vi "AdvancedProgram.vi"() -> ()   [LabVIEW 2018, in "JULABO DeviceDriver.lvlib"]
doc: "Advanced event triggered example"
uses:
  JULABO DeviceDriver.lvlib
panel:
  out "device error out":errorcluster
  out "error out 2":errorcluster caption="error out"
  out "error out":errorcluster
  in  "Registerkartenelement":T1(tab)
  out "Safetytemp":dbl
  out "ExcessTempProtection":dbl
  in  "Control":enum16{"Internal", "External"}(ring)
  out "ExternalTemp":dbl format="%.2f"
  in  "Setpoint":dbl format="%.2f"
  out "InternalTemp":dbl format="%.2f"
  out "Power":i8(slide) scale=-100.0..100.0
  out "Diagram":T2(graph)
  in  "StartStop":bool
  in  "btnAdjustInternalTempLimits":bool
  in  "btnAdjustBandLimits":bool
  in  "btnAdjustCapacityLevels":bool
  in  "btnAdjustWarningLevels":bool
  in  "Upper Bandlimit":dbl=100.0 min=0.0 max=200.0
  in  "Lower Bandlimit":dbl min=0.0 max=200.0
  in  "InternMin":dbl format="%.2f"
  in  "InternMax":dbl=50.0 format="%.2f"
  in  "CoolMax":i8=-100 min=-100 max=0
  in  "HeatMax":u8=50 max=100
  in  "Subtemp":dbl=-20.0 format="%.2f"
  in  "Overtemp":dbl=50.0 format="%.2f"
  in  "Tv (0s) 2":u16 max=999
  in  "Tn (3s) 2":u16=3 min=3 max=9999
  in  "Xp (0.6K) 2":dbl=0.6 min=0.1 max=99.9
  in  "btnAdjustExternalControlParams":bool
  in  "XpU (0.6K)":dbl=0.6 min=0.1 max=99.9
  in  "Dynamic (0: aperiodic)":enum16{"aperiodic", "standard"}(ring)
  in  "btnAdjustInternalControlParams":bool
  in  "Tv (0s)":u16 max=999
  in  "Tn (3s)":u16=3 min=3 max=9999
  in  "Xp (0.6K)":dbl=0.6 min=0.1 max=99.9
  in  "ReadCycle":i32=1000
  in  "Stopp":bool
  in  "ID Query? (T: Yes)":bool=TRUE
  in  "RS485-Address (128: RS232)":u32=128
  in  "VISA resource name":refnum<visa-resource-name>="COM3"
  in  "Serial Configuration":T3={"Baud Rate"=4800, "Parity"=2, "Data Bits"=7, "Stop Bits"=10, "Flow Control"=2} {"Flow Control" items=["None", "XON/XOFF", "RTS/CTS", "XON/XOFF & RTS/CTS", "DTR/DSR", "XON/XOFF & DTR/DSR"]; "Stop Bits" items=["1.0"=10, "1.5"=15, "2.0"=20]; "Data Bits" items=["7"=7, "8"=8]; "Parity" items=["None", "Odd", "Even", "Mark", "Space"]; "Baud Rate" items=["300"=300, "600"=600, "1200"=1200, "2400"=2400, "4800"=4800, "9600"=9600, "19200"=19200]}
  in  "Reset / Default (T: Both)":bool=TRUE
  # "1. Select the COM-Port and adjust the serial\nconfiguration for your instrument\n2. Adjust the Read cycle\n3. Start the VI by pressing the \"Start\" -Button\n( Arrow button on the top-left corner)\n4. To stop the execution press the \"Stop\" button"
  # "Internal parameters"
  # "External parameters"
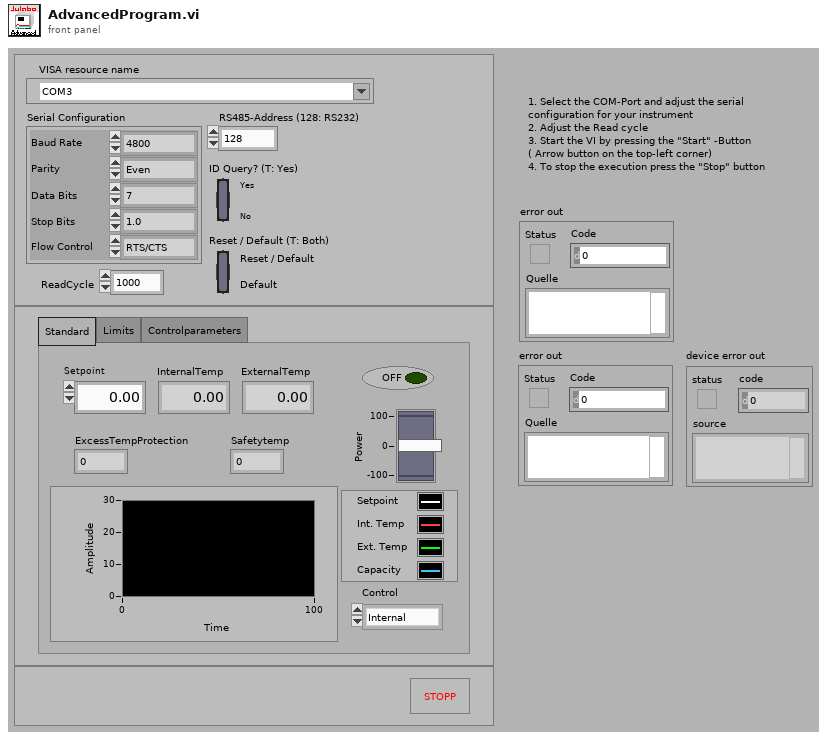
[diagram p1: front panel]
types:
  T1 = enum32{"Standard", "Limits", "Controlparameters"}
  T2 = cluster{"Setpoint (out)":dbl, "InternalTemp (out)":dbl, "ExternalTemp (out)":dbl, "Capacity (out)":i8}
  T3 = cluster{"Baud Rate":u32, "Parity":u16, "Data Bits":u16, "Stop Bits":u16, "Flow Control":u16}
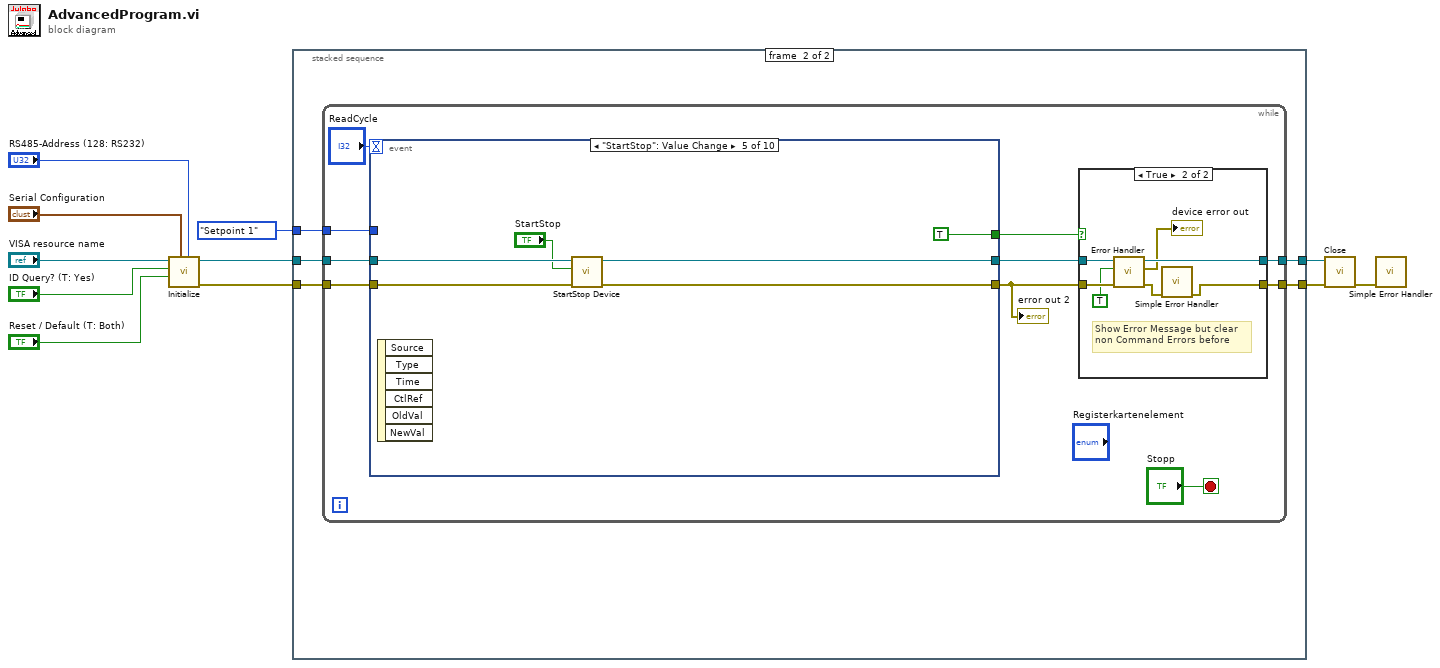
[diagram p0: block diagram]
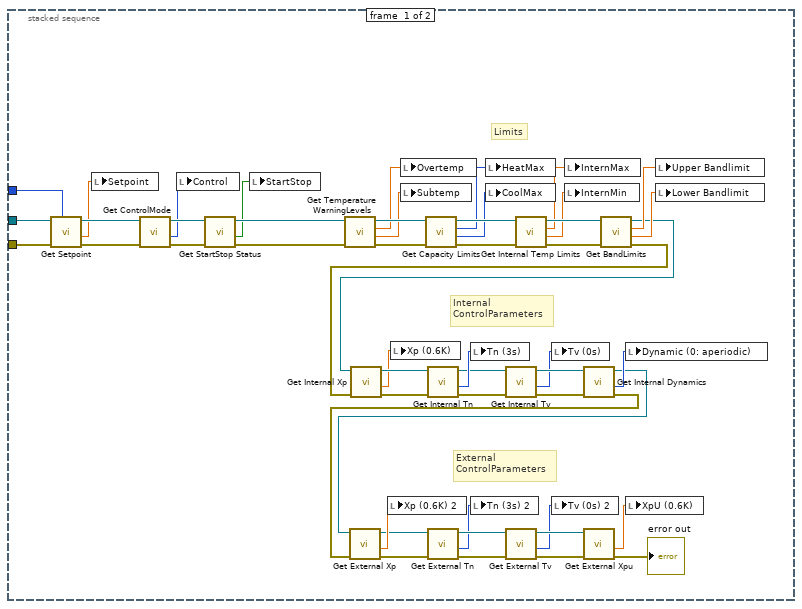
[diagram p2: hidden frame]
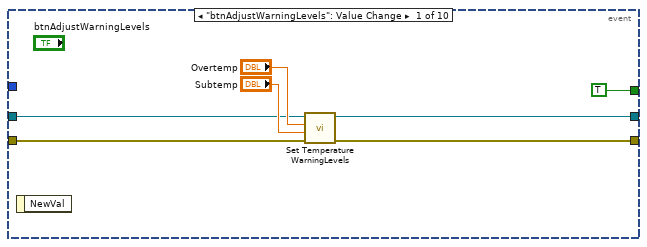
[diagram p4: hidden frame]
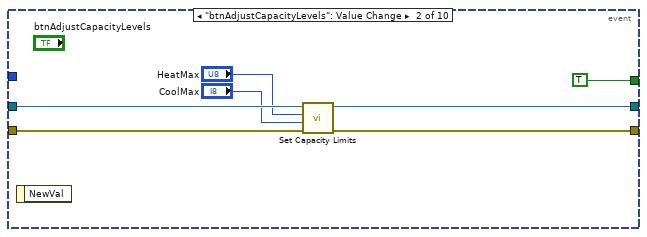
[diagram p5: hidden frame]
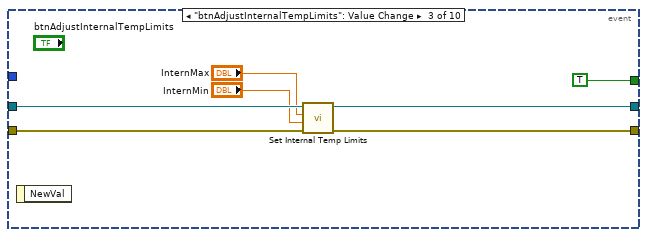
[diagram p6: hidden frame]
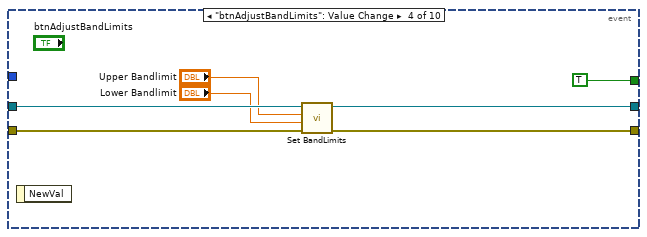
[diagram p7: hidden frame]
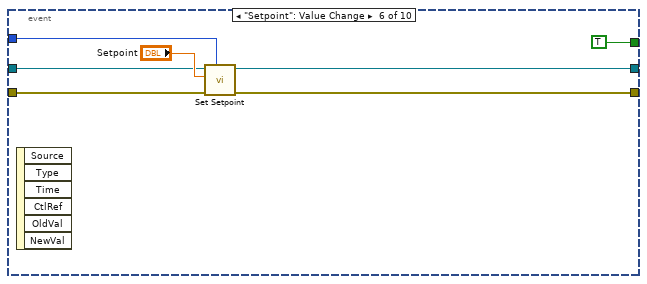
[diagram p8: hidden frame]
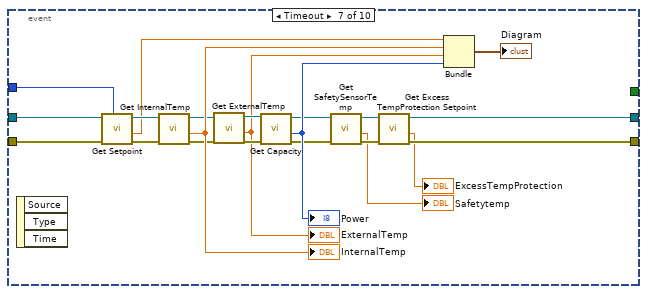
[diagram p9: hidden frame]
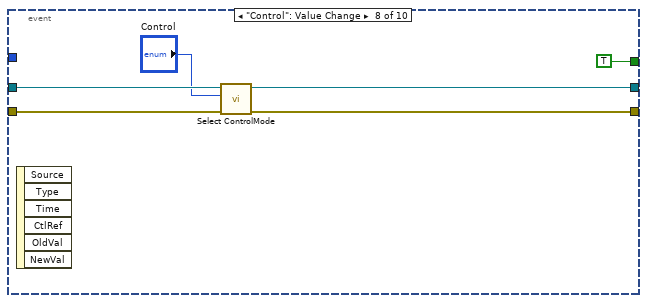
[diagram p10: hidden frame]
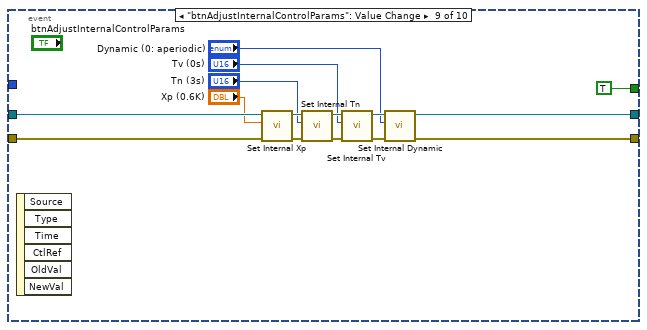
[diagram p11: hidden frame]
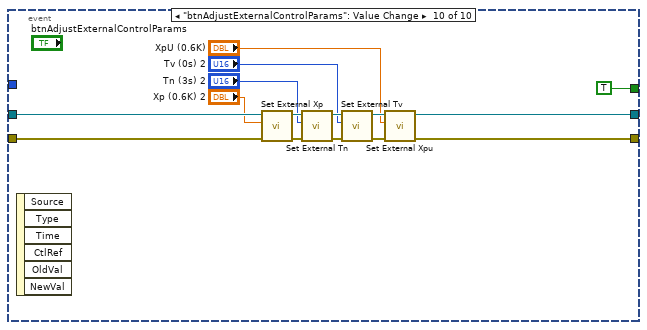
[diagram p12: hidden frame]
diagram:
  n1 = call "Initialize.vi"("RS485-Address (128: RS232)"="RS485-Address (128: RS232)", "Serial Configuration"="Serial Configuration", "Reset / Default (T: Both)"="Reset / Default (T: Both)", "ID Query? (T: Yes)"="ID Query? (T: Yes)", "VISA resource name"="VISA resource name") -> ("error out"=w4:errorcluster, "VISA resource name out"=w5:refnum<visa-resource-name>)  [unwired: 5 in]
  n2 = stacked-sequence {
    tunnel: w5 -> [w17 w67]
    tunnel: w4 -> [w16 w66]
    tunnel: [_ w65] -> w3
    tunnel: [_ w64] -> w2
    tunnel: enum16{"Setpoint 1", "Setpoint 2", "Setpoint 3"}."Setpoint 1" ("Setpointindex") -> [w13 w63]
    frame #0 {
      # "External\nControlParameters"
      # "Internal\nControlParameters"
      # "Limits"
      n3 = call "Get Setpoint.vi"("Setpointindex"=w13, "error in (no error)"=w16, "VISA resource name"=w17) -> ("error out"=w14:errorcluster, "Setpoint (out)"=w12:dbl, "VISA resource name out"=w15:refnum<visa-resource-name>)  [unwired: 6 in]
      n4 = local write "Setpoint"(w12) -> ()
      n5 = call "Get ControlMode.vi"("error in"=w14, "VISA resource name in"=w15) -> ("error out"=w19:errorcluster, "Control (out)"=w23:enum16{"Internal", "External"}, "VISA resource name out"=w24:refnum<visa-resource-name>)  [unwired: 7 in]
      n6 = local write "Control"(w23) -> ()
      n7 = call "Get StartStop Status.vi"("error in"=w19, "VISA resource name in"=w24) -> ("error out"=w18:errorcluster, "Status"=w20:bool, "VISA resource name out"=w21:refnum<visa-resource-name>)  [unwired: 7 in]
      n8 = local write "StartStop"(w20) -> ()
      n9 = call "Get Temperature WarningLevels.vi"("error in (no error)"=w18, "VISA resource name"=w21) -> ("error out"=w59:errorcluster, "Subtemp (out)"=w50:dbl, "Overtemp (out)"=w49:dbl, "VISA resource name out"=w62:refnum<visa-resource-name>)  [unwired: 2 in]
      n10 = local write "Overtemp"(w49) -> ()
      n11 = local write "Subtemp"(w50) -> ()
      n12 = call "Get Capacity Limits.vi"("error in (no error)"=w59, "VISA resource name"=w62) -> ("error out"=w58:errorcluster, "Maximum cooling capacity(out)"=w52:i8, "Maximum heating capacity(out)"=w51:u8, "VISA resource name out"=w61:refnum<visa-resource-name>)  [unwired: 2 in]
      n13 = local write "HeatMax"(w51) -> ()
      n14 = local write "CoolMax"(w52) -> ()
      n15 = call "Get Internal Temp Limits.vi"("error in (no error)"=w58, "VISA resource name"=w61) -> ("error out"=w57:errorcluster, "IntMin (out)"=w54:dbl, "IntMax (out)"=w53:dbl, "VISA resource name out"=w60:refnum<visa-resource-name>)  [unwired: 2 in]
      n16 = local write "InternMax"(w53) -> ()
      n17 = local write "InternMin"(w54) -> ()
      n18 = call "Get BandLimits.vi"("error in (no error)"=w57, "VISA resource name"=w60) -> ("error out"=w37:errorcluster, "LowerBand (out)"=w56:dbl, "UpperBand (out)"=w55:dbl, "VISA resource name out"=w38:refnum<visa-resource-name>)  [unwired: 2 in]
      n19 = call "Get Internal Xp.vi"("error in"=w37, "VISA resource name in"=w38) -> ("error out"=w40:errorcluster, "InternalXp (out)"=w39:dbl, "VISA resource name out"=w41:refnum<visa-resource-name>)  [unwired: 7 in]
      n20 = local write "Xp (0.6K)"(w39) -> ()
      n21 = call "Get Internal Tn.vi"("error in"=w40, "VISA resource name in"=w41) -> ("error out"=w42:errorcluster, "InternalTn (out)"=w48:u16, "VISA resource name out"=w43:refnum<visa-resource-name>)  [unwired: 7 in]
      n22 = local write "Tn (3s)"(w48) -> ()
      n23 = call "Get Internal Tv.vi"("error in"=w42, "VISA resource name in"=w43) -> ("error out"=w45:errorcluster, "InternalTv (out)"=w44:u16, "VISA resource name out"=w46:refnum<visa-resource-name>)  [unwired: 7 in]
      n24 = local write "Tv (0s)"(w44) -> ()
      n25 = call "Get Internal Dynamics.vi"("error in"=w45, "VISA resource name in"=w46) -> ("error out"=w29:errorcluster, "Dynamic (out)"=w47:enum16{"aperiodic", "standard"}, "VISA resource name out"=w28:refnum<visa-resource-name>)  [unwired: 7 in]
      n26 = call "Get External Xp.vi"("error in"=w29, "VISA resource name in"=w28) -> ("error out"=w32:errorcluster, "ExternalXp (out)"=w31:dbl, "VISA resource name out"=w27:refnum<visa-resource-name>)  [unwired: 7 in]
      n27 = local write "Xp (0.6K) 2"(w31) -> ()
      n28 = call "Get External Tn.vi"("error in"=w32, "VISA resource name in"=w27) -> ("error out"=w36:errorcluster, "ExternalTn (out)"=w26:u16, "VISA resource name out"=w35:refnum<visa-resource-name>)  [unwired: 7 in]
      n29 = local write "Tn (3s) 2"(w26) -> ()
      n30 = call "Get External Tv.vi"("error in"=w36, "VISA resource name in"=w35) -> ("error out"=w34:errorcluster, "ExternalTv (out)"=w25:u16, "VISA resource name out"=w33:refnum<visa-resource-name>)  [unwired: 7 in]
      n31 = local write "Tv (0s) 2"(w25) -> ()
      n32 = call "Get External Xpu.vi"("error in"=w34, "VISA resource name in"=w33) -> ("error out"=→"error out":errorcluster, "ExternalXpu (out)"=w30:dbl)  [unwired: 7 in, 1 out]
      n33 = local write "Dynamic (0: aperiodic)"(w47) -> ()
      n34 = local write "XpU (0.6K)"(w30) -> ()
      n35 = local write "Upper Bandlimit"(w55) -> ()
      n36 = local write "Lower Bandlimit"(w56) -> ()
    }
    frame #1 {
      n37 = while {
        tunnel: w67 -> [w77]
        tunnel: w66 -> [w76]
        tunnel: [w74] -> w64
        tunnel: [w73] -> w65
        tunnel: w63 -> [w69]
        stop <- "Stopp" stop-if-true
        n38 = event shown="[4] \"StartStop\": Value Change" {
          selector: _ -> [_ _ _ _ _ _ _ _ _ _]
          dyn-events: _ -> [_ _ _ _ _ _ _ _ _ _]
          timeout: "ReadCycle" -> [_ _ _ _ _ _ _ _ _ _]
          tunnel: [w88 w96 w106 w113 w117 w124 w134 w153 w159 w174] -> w75
          tunnel: [w87 w95 w105 w112 w118 w123 w133 w152 w157 w172] -> w68
          tunnel: w77 -> [w91 w100 w104 w110 w116 w126 w145 w155 w170 w185]
          tunnel: w76 -> [w90 w99 w103 w111 w119 w125 w144 w154 w169 w184]
          tunnel: [TRUE TRUE TRUE TRUE TRUE TRUE _ TRUE TRUE TRUE] -> w72
          tunnel: w69 -> [_ _ _ _ _ w121 w128 _ _ _]
          event "btnAdjustWarningLevels": Value Change {
            n39 = event-data() -> ()  [unwired: 1 in, 1 out]
            n40 = call "Set Temperature WarningLevels.vi"("error in (no error)"=w90, "Subtemp (-20.00°C)"="Subtemp", "Overtemp (50.00°C)"="Overtemp", "VISA resource name"=w91) -> ("error out"=w87:errorcluster, "VISA resource name out"=w88:refnum<visa-resource-name>)  [unwired: 6 in]
          }
          event "btnAdjustCapacityLevels": Value Change {
            n41 = event-data() -> ()  [unwired: 1 in, 1 out]
            n42 = call "Set Capacity Limits.vi"("error in (no error)"=w99, "Maximum cooling capacity(-100%)"="CoolMax", "Maximum heating capacity(100%)"="HeatMax", "VISA resource name"=w100) -> ("error out"=w95:errorcluster, "VISA resource name out"=w96:refnum<visa-resource-name>)  [unwired: 6 in]
          }
          event "btnAdjustInternalTempLimits": Value Change {
            n43 = event-data() -> ()  [unwired: 1 in, 1 out]
            n44 = call "Set Internal Temp Limits.vi"("error in (no error)"=w103, "InternMin (-20.00 °C)"="InternMin", "InternMax (50.00 °C)"="InternMax", "VISA resource name"=w104) -> ("error out"=w105:errorcluster, "VISA resource name out"=w106:refnum<visa-resource-name>)  [unwired: 6 in]
          }
          event "btnAdjustBandLimits": Value Change {
            n45 = event-data() -> ()  [unwired: 1 in, 1 out]
            n46 = call "Set BandLimits.vi"("error in (no error)"=w111, "Lower Bandlimit (200K)"="Lower Bandlimit", "Upper Bandlimit (200K)"="Upper Bandlimit", "VISA resource name"=w110) -> ("error out"=w112:errorcluster, "VISA resource name out"=w113:refnum<visa-resource-name>)  [unwired: 6 in]
          }
          event "StartStop": Value Change {
            n47 = event-data() -> ()  [unwired: 1 in, 6 out]
            n48 = call "StartStop Device.vi"("error in (no error)"=w119, "Start/Stop (f:Stop)"="StartStop", "VISA resource name"=w116) -> ("error out"=w118:errorcluster, "VISA resource name out"=w117:refnum<visa-resource-name>)  [unwired: 7 in]
          }
          event "Setpoint": Value Change {
            n49 = event-data() -> ()  [unwired: 1 in, 6 out]
            n50 = call "Set Setpoint.vi"("Setpointindex (Setpoint1: Default)"=w121, "error in (no error)"=w125, "newSetpoint (20.00°C)"="Setpoint", "VISA resource name"=w126) -> ("error out"=w123:errorcluster, "VISA resource name out"=w124:refnum<visa-resource-name>)  [unwired: 6 in]
          }
          event Timeout {
            n51 = event-data() -> ()  [unwired: 1 in, 3 out]
            n52 = call "Get Setpoint.vi"("Setpointindex"=w128, "error in (no error)"=w144, "VISA resource name"=w145) -> ("error out"=w149:errorcluster, "Setpoint (out)"=w143:dbl, "VISA resource name out"=w148:refnum<visa-resource-name>)  [unwired: 6 in]
            n53 = call "Get InternalTemp.vi"("error in (no error)"=w149, "VISA resource name"=w148) -> ("error out"=w141:errorcluster, "InternalTemp (out)"=w146:dbl, "VISA resource name out"=w142:refnum<visa-resource-name>)  [unwired: 7 in]
            "InternalTemp" <- w146
            n54 = call "Get ExternalTemp.vi"("error in (no error)"=w141, "VISA resource name"=w142) -> ("error out"=w139:errorcluster, "ExternalTemp (out)"=w137:dbl, "VISA resource name out"=w140:refnum<visa-resource-name>)  [unwired: 6 in, 1 out]
            "ExternalTemp" <- w137
            n55 = call "Get Capacity.vi"("error in (no error)"=w139, "VISA resource name"=w140) -> ("error out"=w131:errorcluster, "Capacity (out)"=w138:i8, "VISA resource name out"=w136:refnum<visa-resource-name>)  [unwired: 7 in]
            "Power" <- w138
            n56 = call "Get SafetySensorTemp.vi"("error in (no error)"=w131, "VISA resource name"=w136) -> ("error out"=w132:errorcluster, "Safetytemp (out)"=→"Safetytemp":dbl, "VISA resource name out"=w135:refnum<visa-resource-name>)  [unwired: 7 in]
            n57 = call "Get Excess TempProtection Setpoint.vi"("error in (no error)"=w132, "VISA resource name"=w135) -> ("error out"=w133:errorcluster, "ExcessTempProtection(out)"=→"ExcessTempProtection":dbl, "VISA resource name out"=w134:refnum<visa-resource-name>)  [unwired: 7 in]
            n58 = Bundle("Setpoint (out)"=w143, "InternalTemp (out)"=w146, "ExternalTemp (out)"=w137, "Capacity (out)"=w138) -> (→"Diagram":T2)  [unwired: 1 in]
          }
          event "Control": Value Change {
            n59 = event-data() -> ()  [unwired: 1 in, 6 out]
            n60 = call "Select ControlMode.vi"("error in (no error)"=w154, "Control (0: Internal)"="Control", "VISA resource name"=w155) -> ("error out"=w152:errorcluster, "VISA resource name out"=w153:refnum<visa-resource-name>)  [unwired: 7 in]
          }
          event "btnAdjustInternalControlParams": Value Change {
            n61 = event-data() -> ()  [unwired: 1 in, 6 out]
            n62 = call "Set Internal Xp.vi"("error in (no error)"=w169, "Xp (0.6K)"="Xp (0.6K)", "VISA resource name"=w170) -> ("error out"=w166:errorcluster, "VISA resource name out"=w165:refnum<visa-resource-name>)  [unwired: 7 in]
            n63 = call "Set Internal Tn.vi"("error in (no error)"=w166, "Tn (3s)"="Tn (3s)", "VISA resource name"=w165) -> ("error out"=w168:errorcluster, "VISA resource name out"=w167:refnum<visa-resource-name>)  [unwired: 7 in]
            n64 = call "Set Internal Tv.vi"("error in (no error)"=w168, "Tv (0s)"="Tv (0s)", "VISA resource name"=w167) -> ("error out"=w158:errorcluster, "VISA resource name out"=w161:refnum<visa-resource-name>)  [unwired: 7 in]
            n65 = call "Set Internal Dynamic.vi"("error in (no error)"=w158, "Dynamic (0: aperiodic)"="Dynamic (0: aperiodic)", "VISA resource name"=w161) -> ("error out"=w157:errorcluster, "VISA resource name out"=w159:refnum<visa-resource-name>)  [unwired: 7 in]
          }
          event "btnAdjustExternalControlParams": Value Change {
            n66 = event-data() -> ()  [unwired: 1 in, 6 out]
            n67 = call "Set External Xp.vi"("error in (no error)"=w184, "Xp (0.6K)"="Xp (0.6K) 2", "VISA resource name"=w185) -> ("error out"=w181:errorcluster, "VISA resource name out"=w180:refnum<visa-resource-name>)  [unwired: 7 in]
            n68 = call "Set External Tn.vi"("error in (no error)"=w181, "Tn (3s)"="Tn (3s) 2", "VISA resource name"=w180) -> ("error out"=w183:errorcluster, "VISA resource name out"=w182:refnum<visa-resource-name>)  [unwired: 7 in]
            n69 = call "Set External Tv.vi"("error in (no error)"=w183, "Tv (0s)"="Tv (0s) 2", "VISA resource name"=w182) -> ("error out"=w173:errorcluster, "VISA resource name out"=w176:refnum<visa-resource-name>)  [unwired: 7 in]
            n70 = call "Set External Xpu.vi"("error in (no error)"=w173, "XpU (0.6K)"="XpU (0.6K)", "VISA resource name"=w176) -> ("error out"=w172:errorcluster, "VISA resource name out"=w174:refnum<visa-resource-name>)  [unwired: 7 in]
          }
        }
        "error out 2" <- w68
        n71 = case shown="True" w72 {
          tunnel: w75 -> [w79 w84]
          tunnel: [w79 w82] -> w74
          tunnel: w68 -> [w78 w85]
          tunnel: [w78 w86] -> w73
          frame False {
          }
          frame True {
            # "Show Error Message but clear\nnon Command Errors before"
            n72 = call "Error Handler.vi"("error in (no error)"=w85, "ClearDeviceError (false)"=TRUE, "VISA resource name"=w84) -> ("error out"=w83:errorcluster, "device error out"=→"device error out":errorcluster, "VISA resource name out"=w82:refnum<visa-resource-name>)  [unwired: 5 in, 1 out]
            n73 = call <vilib>:"Simple Error Handler.vi"("error in (no error)"=w83) -> ("error out"=w86:errorcluster)  [unwired: 4 in, 4 out]
          }
        }
      }
    }
  }
  n74 = call "Close.vi"("error in (no error)"=w3, "VISA resource name"=w2) -> ("error out"=w9:errorcluster)  [unwired: 9 in]
  n75 = call <vilib>:"Simple Error Handler.vi"("error in (no error)"=w9) -> ()  [unwired: 4 in, 5 out]
